vi "Loadbitpattern.vi"() -> ()   [LabVIEW 2011]
panel:
  out "LoadBitPattern":variant
  in  "PLTS.IPLTSApplication":refnum<k7>
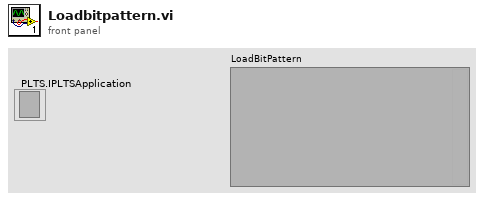
[diagram p1: front panel]
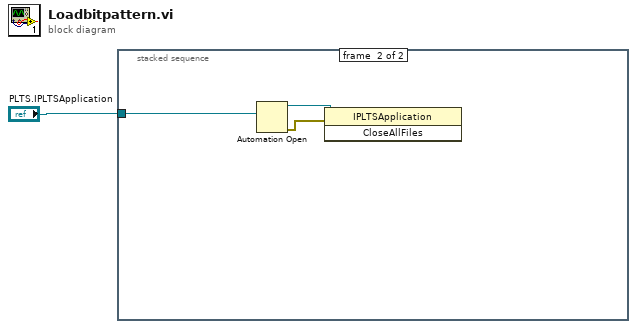
[diagram p0: block diagram]
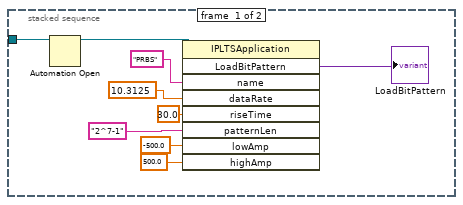
[diagram p2: hidden frame]
diagram:
  n1 = stacked-sequence {
    tunnel: "PLTS.IPLTSApplication" -> [w10 w13]
    frame #0 {
      n2 = Automation Open(Automation Refnum=w10) -> (Automation Refnum=w9:refnum<k7>)  [unwired: 3 in, 1 out]
      n3 = invoke class="IPLTSApplication" method="LoadBitPattern"(reference=w9, "name"="PRBS", "dataRate"=10.3125, "riseTime"=30.0, "patternLen"="2^7-1", "lowAmp"=-500.0, "highAmp"=500.0) -> ("LoadBitPattern"=→"LoadBitPattern":variant)  [unwired: 2 in, 8 out]
    }
    frame #1 {
      n4 = Automation Open(Automation Refnum=w13) -> (Automation Refnum=w12:refnum<k7>, error out=w11:errorcluster)  [unwired: 3 in]
      n5 = invoke class="IPLTSApplication" method="CloseAllFiles"(reference=w12, error in=w11) -> ()  [unwired: 1 in, 3 out]
    }
  }
